vi "WriteIconsTDMS.vi"() -> ()   [LabVIEW 2014]
uses:
  <userlib>/_LAVACR/Scripting Tools/Scripting Tools.lvlib
panel:
  out "IconsFromFile":picture[](array[picture])
  in  "file path":path
  out "Class Hierarchy 2":string[][](array[string])
  out "Labels":string[](array[string])
  out "ClassName":string[](array[string])
  out "ClassName":string[](array[string])
  out "Class Hierarchy":string[][](array[string])
  out "Icons":picture[](array[picture])
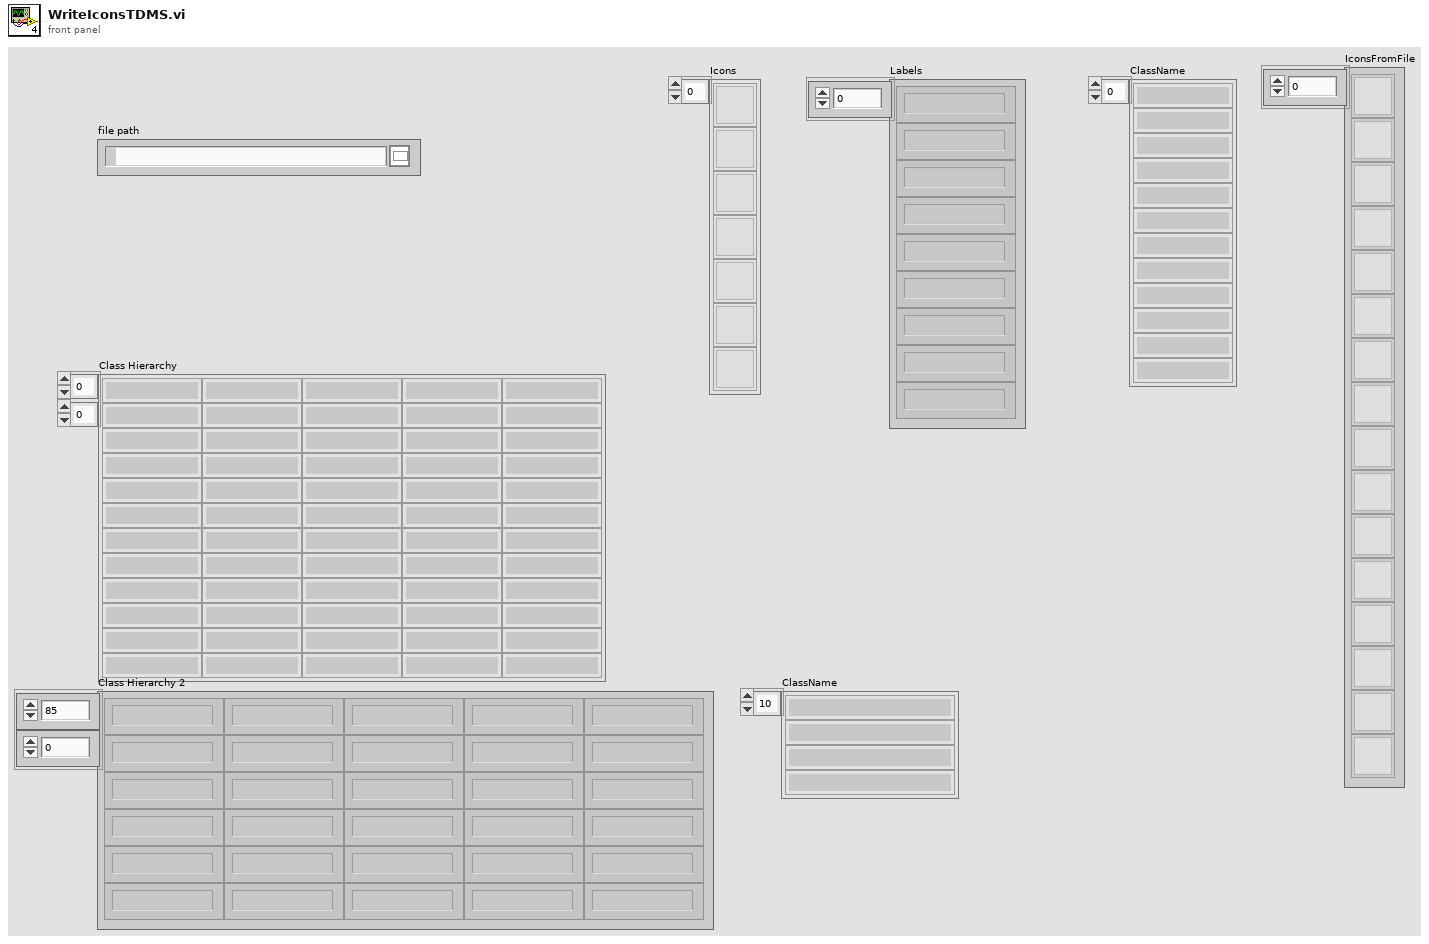
[diagram p1: front panel]
types:
  T1 = enum16{"open", "open or create", "create or replace", "create", "open (read-only)"}
  T2 = typedef "imagedata.ctl" = cluster{"image type":i32, "image depth":i32, "image":u8[], "mask":u8[], "colors":u32[], "Rectangle":cluster{"left":i16, "top":i16, "right":i16, "bottom":i16}}
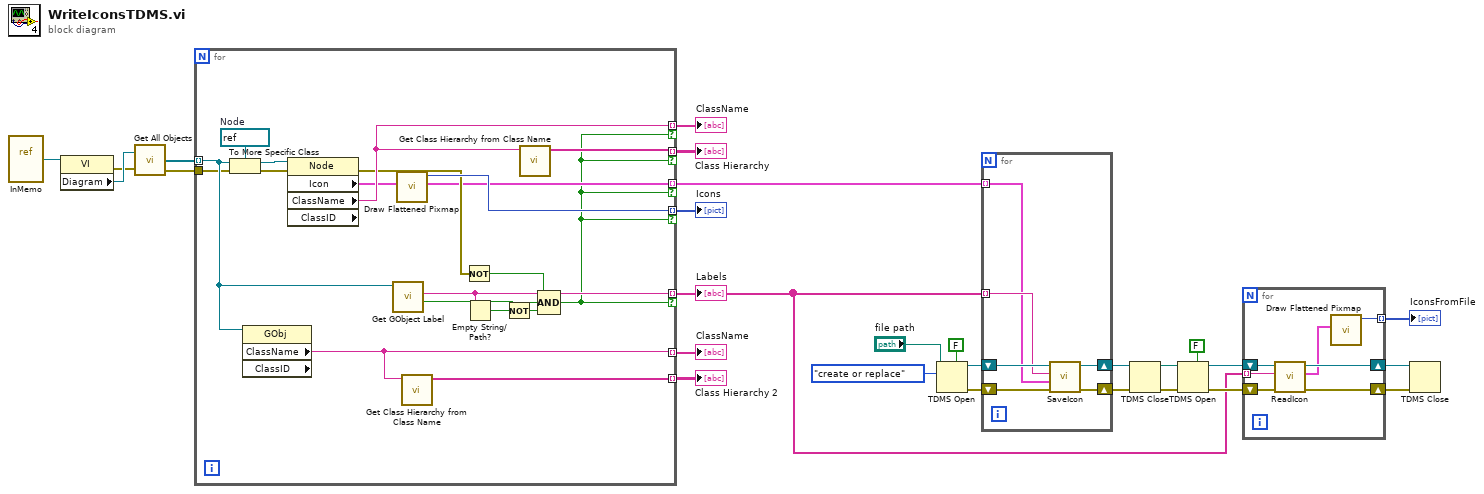
[diagram p0: block diagram]
diagram:
  n1 = vi-ref "InMemo.vi"() -> (w22:refnum<vi>)
  n2 = property class="VI"(reference=w22) -> (error out=w20:errorcluster, "Diagram"=w21:refnum<vi>)  [unwired: 1 in, 1 out]
  n3 = call <userlib>:"Get All Objects.vi"("Diagram In"=w21, "error in"=w20) -> ("All Objects"=w27:refnum<vi>[], "error out"=w19:errorcluster)  [unwired: 1 out]
  n4 = for {
    tunnel: w27 -> [w40] mode=indexing
    tunnel: [w45] -> w26 mode=indexing if=w28
    tunnel: [w42] -> w25 mode=indexing if=w28
    tunnel: [w41] -> w24 mode=indexing if=w28
    tunnel: [w32] -> w23 mode=indexing
    tunnel: [w39] -> w2 mode=indexing if=w28
    tunnel: [w31] -> w18 mode=indexing
    tunnel: w19 -> [w33]
    tunnel: [w29] -> w8 mode=indexing if=w28
    w44 = refnum<vi> refnum  # Node
    n5 = To More Specific Class(target class=w44, reference=w40, error in=w33) -> (specific class reference=w43:refnum<vi>, error out=w30:errorcluster)
    n6 = property class="GObj" props=["ClassName", "ClassID"](reference=w40) -> ("ClassName"=w32:string)  [unwired: 1 in, 3 out]
    n7 = property class="Node" props=["Icon", "ClassName", "ClassID"](reference=w43, error in=w30) -> (error out=w35:errorcluster, "Icon"=w29:T2, "ClassName"=w41:string)  [unwired: 2 out]
    n8 = call <vilib>:"Get GObject Label.vi"("GObject"=w40) -> ("Object Has Label?"=w36:bool, "Object Label"=w39:string)  [unwired: 6 in, 3 out]
    n9 = call <vilib>:"Draw Flattened Pixmap.vi"("image data"=w29) -> ("new picture"=w45:picture)  [unwired: 8 in]
    n10 = call <vilib>:"Get Class Hierarchy from Class Name.vi"("Class Name"=w32) -> ("Class Hierarchy"=w31:string[])  [unwired: 9 in, 1 out]
    n11 = Not(x=w35) -> (.not. x?=w34:bool)
    n12 = Empty String/Path?(string/path=w39) -> (empty?=w38:bool)
    n13 = Not(x=w38) -> (.not. x?=w37:bool)
    n14 = call <vilib>:"Get Class Hierarchy from Class Name.vi"("Class Name"=w41) -> ("Class Hierarchy"=w42:string[])  [unwired: 9 in, 1 out]
    n15 = Compound Arithmetic op=AND(w34, w36, w37) -> (w28:bool)
  }
  "Icons" <- w26
  "Class Hierarchy" <- w25
  "ClassName" <- w24
  "ClassName" <- w23
  "Labels" <- w2
  "Class Hierarchy 2" <- w18
  n16 = TDMS Open(5:FALSE ("create index file? (T)"), 10:T1."create or replace" ("operation (0:open)"), 11:"file path") -> (0:w9:errorcluster, 3:w10:refnum<k34>)  [unwired: 4 in]
  n17 = for {
    tunnel: w2 -> [w48] mode=indexing
    shift-right: [w50] -> w6
    shift-left: w9 -> [w47]
    shift-right: [w49] -> w7
    shift-left: w10 -> [w51]
    tunnel: w8 -> [w46] mode=indexing
    n18 = call "SaveIcon.vi"("error in (no error)"=w47, "Icon"=w46, "Function"=w48, "TdmsIn"=w51) -> ("error out"=w50:errorcluster, "TdmsOuit"=w49:refnum<k34>)  [unwired: 6 in]
  }
  n19 = TDMS Close(8:w6, 11:w7) -> (0:w3:errorcluster, 3:w4:path)
  n20 = TDMS Open(5:FALSE ("create index file? (T)"), 8:w3, 11:w4) -> (0:w12:errorcluster, 3:w13:refnum<k34>)  [unwired: 4 in]
  n21 = for {
    shift-right: [w55] -> w5
    shift-left: w13 -> [w57]
    shift-right: [w58] -> w14
    shift-left: w12 -> [w56]
    tunnel: w2 -> [w54] mode=indexing
    tunnel: [w52] -> w1 mode=indexing
    n22 = call "ReadIcon.vi"("error in (no error)"=w56, "Function"=w54, "TdmsIn"=w57) -> ("error out"=w58:errorcluster, "Icon"=w53:T2, "TdmsOut"=w55:refnum<k34>)  [unwired: 6 in]
    n23 = call <vilib>:"Draw Flattened Pixmap.vi"("image data"=w53) -> ("new picture"=w52:picture)  [unwired: 8 in]
  }
  "IconsFromFile" <- w1
  n24 = TDMS Close(8:w14, 11:w5) -> ()  [unwired: 2 out]
